vi "Set Offset.vi"(8 "error in (no error)":errorcluster, 10 "Offset":dbl, 11 "CAN Signal in":refnum<class "CAN Signal.lvclass">) -> (0 "error out":errorcluster, 3 "CAN Signal out":refnum<class "CAN Signal.lvclass">)   [LabVIEW 2023, in "CAN Signal.lvclass"]
uses:
  CAN Signal.lvclass
  CAN Signal.lvclass/CAN Signal.ctl
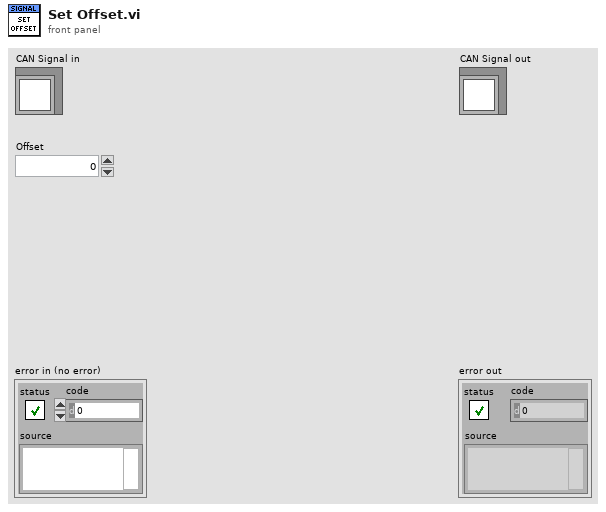
[diagram p1: front panel]
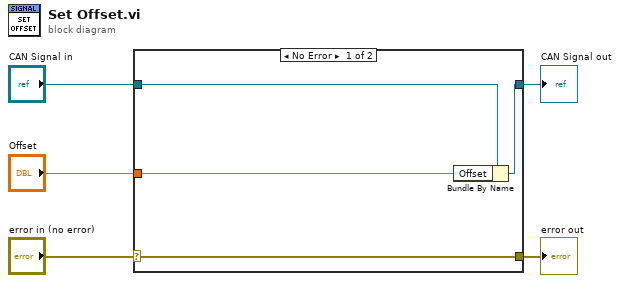
[diagram p0: block diagram]
diagram:
  n1 = case shown="No Error" "error in (no error)" {
    selector: "error in (no error)" -> [w9 w10]
    tunnel: [w9 w10] -> w4
    tunnel: [w7 w11] -> w2
    tunnel: "CAN Signal in" -> [w8 w11]
    tunnel: "Offset" -> [w6 _]
    frame No Error {
      n2 = Bundle By Name(cluster=w8, "Offset"=w6) -> (w7:refnum<class "CAN Signal.lvclass">)
    }
    frame Error {
    }
  }
  "error out" <- w4
  "CAN Signal out" <- w2
